vi "LimelightInterface.vi"(4 "LimeLightActivate":bool, 5 "CameraMounting":T2) -> (0 "TurretAngle(deg)":dbl, 1 "TurretDistance(in)":dbl, 2 "VisionTarget":T1)   [LabVIEW 2019]
uses:
  TypeDefs/ConfigComponents/Config_CameraMounting.ctl
  TypeDefs/VisionTarget.ctl
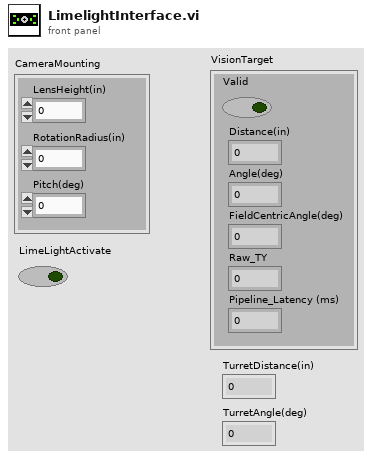
[diagram p1: front panel]
types:
  T1 = typedef "VisionTarget.ctl" = cluster{"Valid":bool, "Distance(in)":dbl, "Angle(deg)":dbl, "FieldCentricAngle(deg)":dbl, "Raw_TY":dbl, "Pipeline_Latency (ms)":dbl}
  T2 = typedef "Config_CameraMounting.ctl" = cluster{"LensHeight(in)":dbl, "RotationRadius(in)":dbl, "Pitch(deg)":dbl}
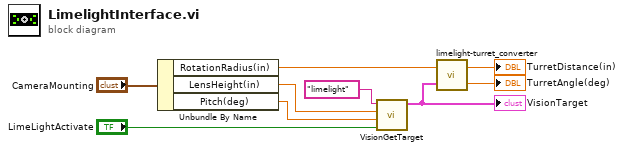
[diagram p0: block diagram]
diagram:
  n1 = Unbundle By Name("CameraMounting") -> ("RotationRadius(in)"=w6:dbl, "LensHeight(in)"=w8:dbl, "Pitch(deg)"=w7:dbl)
  n2 = call "VisionGetTarget.vi"("LimelightActivate"="LimeLightActivate", "Camera Pitch [deg.]"=w7, "Camera Height[in.]"=w8, "Limelight name"="limelight") -> ("VisionTarget"=w1:T1)  [unwired: 7 in]
  "VisionTarget" <- w1
  n3 = call "limelight-turret_converter.vi"("VisionTarget"=w1, "Limelight Radius (in)"=w6) -> ("Turret Yaw Angle (deg)"=→"TurretAngle(deg)":dbl, "Turret Distance (in)"=→"TurretDistance(in)":dbl)
